vi "Color Box Example.vi"() -> ()   [LabVIEW 2009]
panel:
  in  "Slide":dbl(slide) scale=0.0..250.0
  out "Color Box":u32(colorbox)
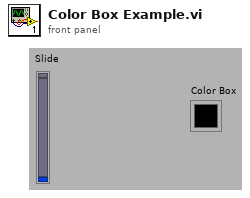
[diagram p1: front panel]
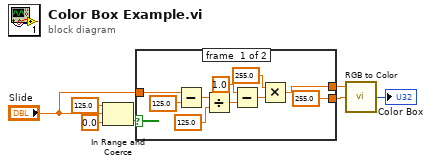
[diagram p0: block diagram]
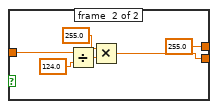
[diagram p2: hidden frame]
diagram:
  n1 = In Range and Coerce(upper limit=125.0, x="Slide", lower limit=0.0) -> (In Range?=w4:bool)  [unwired: 1 out]
  n2 = case shown="False" w4 {
    tunnel: [w17 255.0] -> w1
    tunnel: [255.0 w18] -> w2
    tunnel: "Slide" -> [w14 w21]
    frame #0 {
      n3 = Subtract(x=w14, y=125.0) -> (x-y=w13:dbl)
      n4 = Divide(x=w13, y=125.0) -> (x/y=w11:dbl)
      n5 = Subtract(x=1.0, y=w11) -> (x-y=w9:dbl)
      n6 = Multiply(x=255.0, y=w9) -> (x*y=w17:dbl)
    }
    frame #1 {
      n7 = Divide(x=w21, y=124.0) -> (x/y=w19:dbl)
      n8 = Multiply(x=255.0, y=w19) -> (x*y=w18:dbl)
    }
  }
  n9 = call <vilib>:"RGB to Color.vi"("G"=w2, "R"=w1) -> ("Color"=→"Color Box":u32)  [unwired: 1 in]
